vi "ADD_BIN.vi"(10 "Array":bool[](array[boolean])) -> (2 "SUM":i16)   [LabVIEW 2022 SP3]
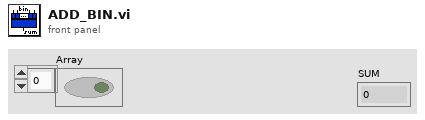
[diagram p1: front panel]
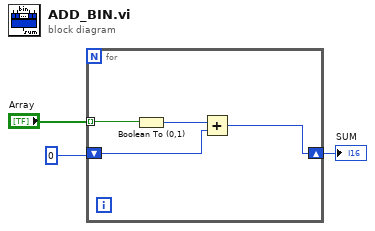
[diagram p0: block diagram]
diagram:
  n1 = for {
    tunnel: "Array" -> [w7] mode=indexing
    shift-right: [w4] -> w1
    shift-left: i16 0 ("0, 1") -> [w5]
    n2 = Boolean To (0,1)(Boolean=w7) -> (0, 1=w6:i16)
    n3 = Add(x=w6, y=w5) -> (x+y=w4:i16)
  }
  "SUM" <- w1
